vi "PVCAM_SetupCont.vi"(0 "hCam":i16, 5 "rgn_total":i16, 7 "rgn_type":T2={"s1"=0, "s2"=1199, "sbin"=1, "p1"=0, "p2"=1199, "pbin"=1}, 9 "exp_mode":i16, 11 "error in (no error)":errorcluster, 12 "exp_time":u32=10, 13 "circ_mode":T1(ring)) -> (4 "stream_size":u32, 6 "return type":i16, 15 "error out":errorcluster)   [LabVIEW 2021]
uses:
  PVCAM_rgn_type.ctl
  pvcam64.dll
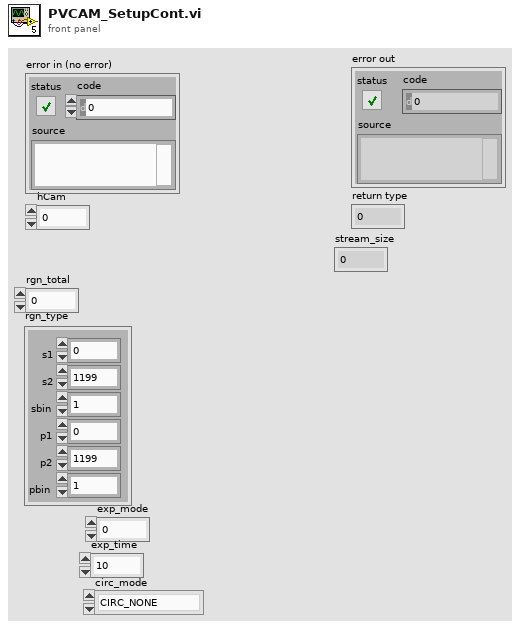
[diagram p1: front panel]
types:
  T1 = enum16{"CIRC_NONE", "CIRC_OVERWRITE", "CIRC_NO_OVERWRITE"}
  T2 = typedef "PVCAM_rgn_type.ctl" = cluster{"s1":u16, "s2":u16, "sbin":u16, "p1":u16, "p2":u16, "pbin":u16}
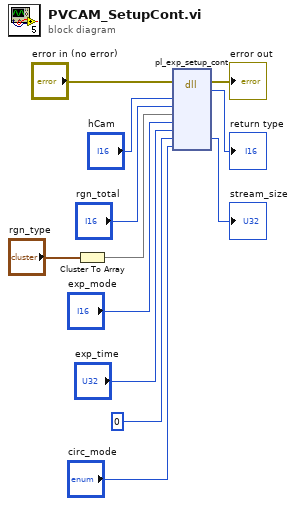
[diagram p0: block diagram]
diagram:
  n1 = Cluster To Array(cluster="rgn_type") -> (array=w7:u16[])
  n2 = dll-call lib="pvcam64.dll" fn="pl_exp_setup_cont"(error in="error in (no error)", "hCam"="hCam", "rgn_total"="rgn_total", "region"=w7, "exp_mode"="exp_mode", "exp_time"="exp_time", "stream_size"=u32 0, "circ_mode"="circ_mode") -> (error out=→"error out":errorcluster, "return type"=→"return type":i16, "stream_size"=→"stream_size":u32)  [unwired: 8 in, 1 out]
